vi "test_alignLeftValidation.vi"(11 "Test Case In":refnum<class "AlignmentTests.lvclass">) -> (0 "error out":errorcluster, 3 "Test Case Out":refnum<class "AlignmentTests.lvclass">)   [LabVIEW 2023, in "AlignmentTests.lvclass"]
uses:
  AlignmentTests.lvclass
  C:/Program Files (x86)/National Instruments/LabVIEW 2023/vi.lib/Astemes/LUnit/Test Case.lvclass
  <vilib>/Astemes/LUnit/Test Case.lvclass/Test Case.ctl
  <vilib>/Astemes/LUnit/Core/LUnit Test Case/Private/Append Pass Result.vi
  <vilib>/Astemes/LUnit/Core/LUnit Test Case/Private/Append Fail Result.vi
  4993e8ee-a06a-463a-9684-69129f64d5ce.vi/9c5d11cd-9439-4240-a1ee-d9baace9c924.vi
  <vilib>/Astemes/LUnit/Core/LUnit Test Case/Private/Run In UI.vi
  <vilib>/Utility/error.llb/Clear Errors.vi
  AlignmentTests.lvclass/AlignmentTests.ctl
  source/TLC_Geometry.lvlib
  <vilib>/Astemes/LUnit/Test Case.lvclass
  C:/Program Files (x86)/National Instruments/LabVIEW 2023/vi.lib/Astemes/LUnit/LUnit Runnable.lvclass
  C:/projects/TLC_Geometry/tests/AlignmentTests/AlignmentTests.lvclass
panel:
  in  "Numeric 3":dbl
  in  "Numeric 2":dbl
  in  "Numeric":dbl
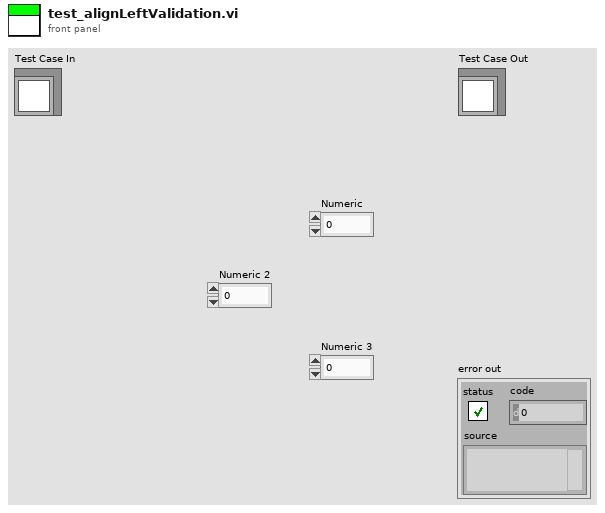
[diagram p1: front panel]
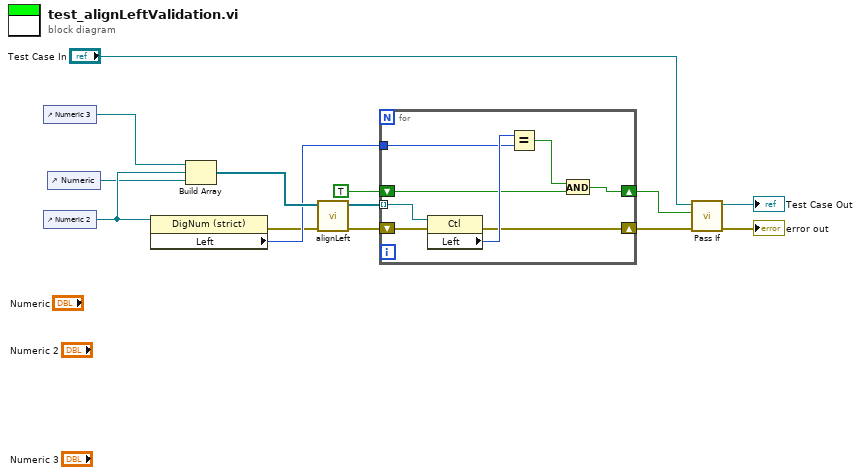
[diagram p0: block diagram]
diagram:
  n1 = control-ref of="Numeric 3"() -> (w11:refnum<vi>)
  n2 = control-ref of="Numeric 2"() -> (w10:refnum<vi>)
  n3 = control-ref of="Numeric"() -> (w9:refnum<vi>)
  n4 = property class="DigNum (strict)"(reference=w10) -> (error out=w1:errorcluster, "Left"=w6:i32)  [unwired: 1 in, 1 out]
  n5 = Build Array(w11, w10, w9) -> (w8:refnum<vi>[])
  n6 = call "alignLeft.vi"("error in (no error)"=w1, "refs"=w8) -> ("error out"=w3:errorcluster, "refs(dup)"=w7:refnum<vi>[])  [unwired: 8 in]
  n7 = for {
    tunnel: w7 -> [w22] mode=indexing
    tunnel: w6 -> [w20]
    shift-right: [w18] -> w4
    shift-left: TRUE -> [w17]
    shift-right: [w15] -> w2
    shift-left: w3 -> [w16]
    n8 = property class="Ctl"(reference=w22, error in=w16) -> (error out=w15:errorcluster, "Left"=w21:i32)  [unwired: 1 out]
    n9 = Equal?(x=w21, y=w20) -> (x = y?=w19:bool)
    n10 = And(x=w19, y=w17) -> (x .and. y?=w18:bool)
  }
  n11 = call <vilib>:"Pass If.vi"("error in (no error)"=w2, "Pass?"=w4, "LUnit Test Case In"="Test Case In") -> ("error out"=→"error out":errorcluster, "LUnit Test Case Out"=→"Test Case Out":refnum<class "AlignmentTests.lvclass">)  [unwired: 7 in]
